vi "Write AIParam one.vi"(6 "AIParam":dbl, 8 "error in (no error)":errorcluster, 9 "Param column":i32, 10 "Param number":i32, 11 "AI in":T1) -> (0 "error out":errorcluster, 3 "AI out":T1)   [LabVIEW 2019, in "Inputs.lvlib"]
uses:
  Inputs.lvlib
  Ctl/AI.ctl
  Ctl/AI short.ctl
  Ctl/Parameter State.ctl
panel:
  # "Analog parameters"
  # "Description of analog parameters"
  # "Analog parameters"
  # "Description of analog parameters"
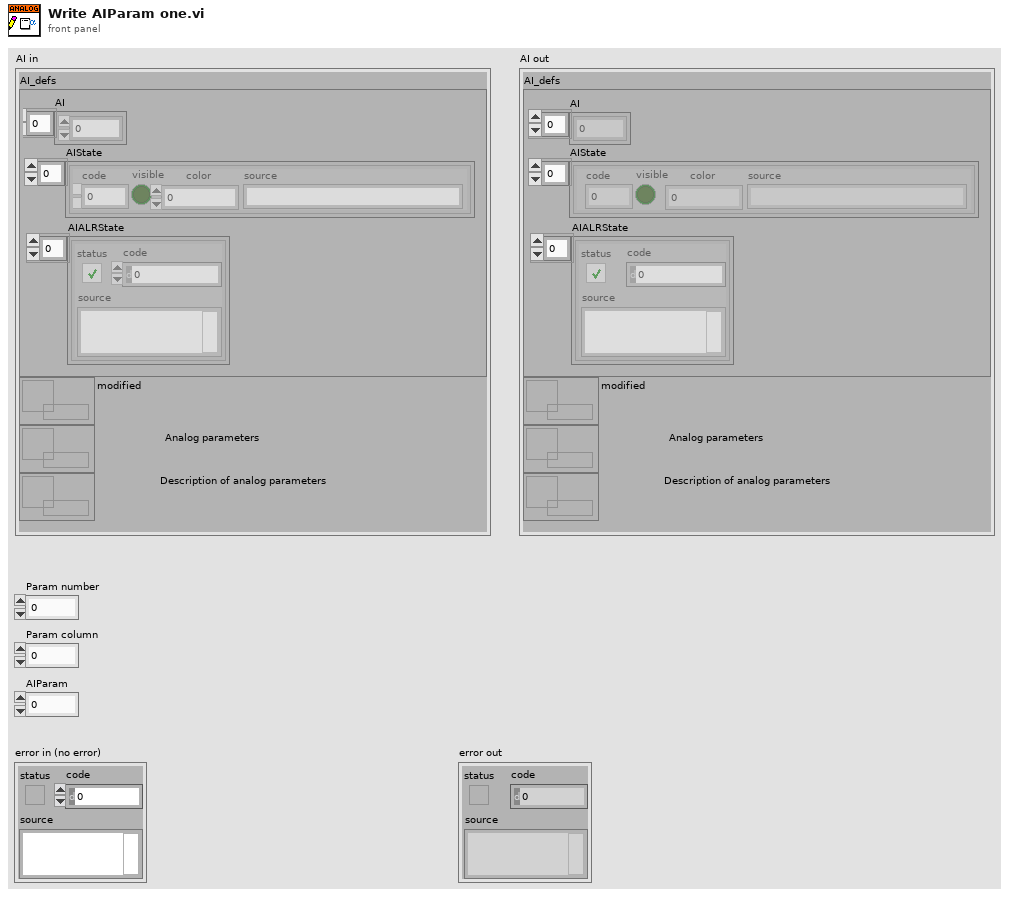
[diagram p1: front panel]
types:
  T1 = typedef "Inputs.lvlib/AI.ctl" = cluster{"AI_defs":T2, "modified":refnum<data-value>, "AIP":refnum<data-value>, "AINames":refnum<data-value>}
  T2 = typedef "Inputs.lvlib/AI short.ctl" = cluster{"AI":dbl[], "AIState":T3[], "AIALRState":errorcluster[]}
  T3 = typedef "Inputs.lvlib/Parameter State.ctl" = cluster{"code":i32, "visible":bool, "color":u32, "source":string}
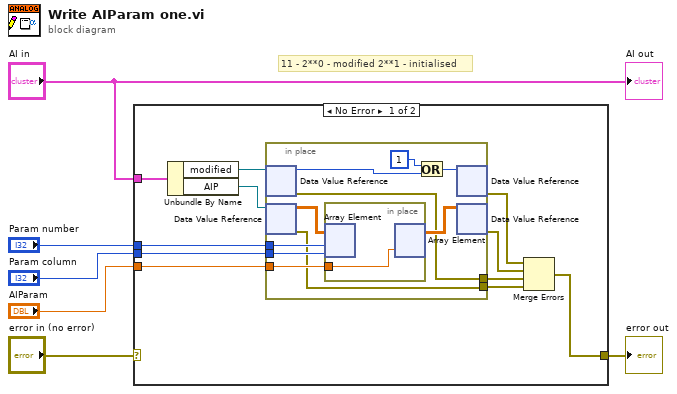
[diagram p0: block diagram]
diagram:
  # "11 - 2**0 - modified 2**1 - initialised"
  n1 = case shown="No Error" "error in (no error)" {
    selector: "error in (no error)" -> [_ w29]
    tunnel: [w16 w29] -> w5
    tunnel: "AI in" -> [w17 _]
    tunnel: "Param number" -> [w14 _]
    tunnel: "Param column" -> [w13 _]
    tunnel: "AIParam" -> [w12 _]
    frame No Error {
      n2 = Unbundle By Name(w17) -> ("modified"=w10:refnum<data-value>, "AIP"=w15:refnum<data-value>)
      n3 = in-place {
        in-place-border: w14 -> [w25]
        in-place-border: w13 -> [w24]
        in-place-border: w12 -> [w23]
        in-place-border: [w22] -> w9
        in-place-border: [w21] -> w8
        n4 = in-place-dvr #1(w10) -> (w19:u8, w21:errorcluster)
        n5 = in-place-dvr #2(w15) -> (w27:dbl[][], w22:errorcluster)
        n6 = in-place {
          in-place-border: w23 -> [w28]
          n7 = in-place-array #3(w27, w25, w24) -> ()  [unwired: 1 out]
          n8 = in-place-array #3(w28) -> (w26:dbl[][])  [unwired: 2 out]
        }
        n9 = Or(x=u8 1 ("data value"), y=w19) -> (x .or. y?=w18:u8)
        n10 = in-place-dvr #1(w18) -> (w7:errorcluster)  [unwired: 1 out]
        n11 = in-place-dvr #2(w26) -> (w11:errorcluster)  [unwired: 1 out]
      }
      n12 = Merge Errors(w7, w11, w8, w9) -> (w16:errorcluster)
    }
    frame Error {
    }
  }
  "error out" <- w5
  "AI out" <- "AI in"
